vi "Send Message.vi"(0 "ICanCommunicate In":refnum<class "ICanCommunicate.lvclass">, 7 "Message":T1, 11 "Error In":errorcluster) -> (4 "ICanCommunicate Out":refnum<class "ICanCommunicate.lvclass">, 15 "Error Out":errorcluster)   [LabVIEW 2023, in "ICanCommunicate.lvclass"]
doc: "Specifies the way of sending messages to other processes."
uses:
  ICanCommunicate.lvclass
  Message.ctl
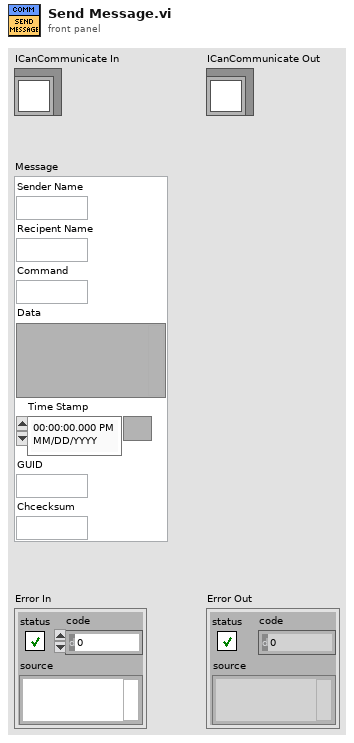
[diagram p1: front panel]
types:
  T1 = typedef "ICanCommunicate.lvclass/Message.ctl" = cluster{"Sender Name":string, "Recipent Name":string, "Command":string, "Data":variant, "Time Stamp":timestamp, "GUID":string, "Chcecksum":string}
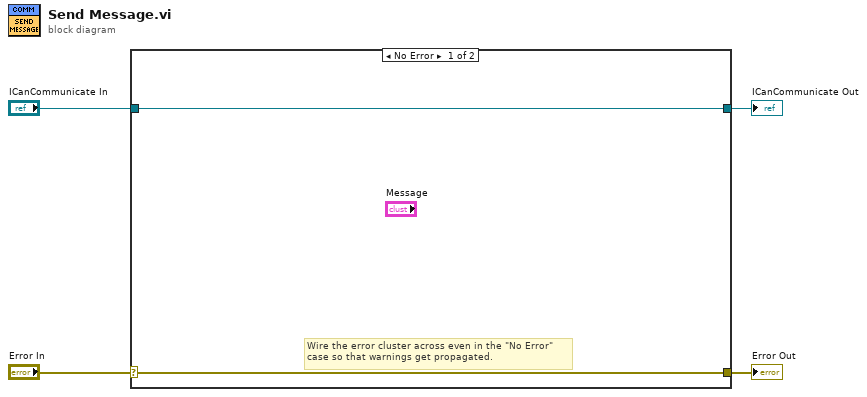
[diagram p0: block diagram]
diagram:
  n1 = case shown="No Error" "Error In" {
    selector: "Error In" -> [w5 w8]
    tunnel: [w5 w8] -> w3
    tunnel: [w6 w7] -> w1
    tunnel: "ICanCommunicate In" -> [w6 w7]
    frame No Error {
      # "Wire the error cluster across even in the \"No Error\"\ncase so that warnings get propagated."
    }
    frame Error {
    }
  }
  "Error Out" <- w3
  "ICanCommunicate Out" <- w1
